vi "Switch.vi"() -> ()   [LabVIEW 2022 SP3]
uses:
  <vilib>/DAQmx/read.llb/DAQmx Read (Digital 1D Bool NChan 1Samp 1Line).vi
  <vilib>/DAQmx/miscellaneous.llb/DAQmx Fill In Error Info.vi
panel:
  out "Switches Bool":bool[](array[boolean])
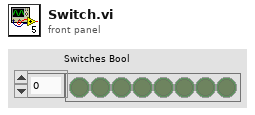
[diagram p1: front panel]
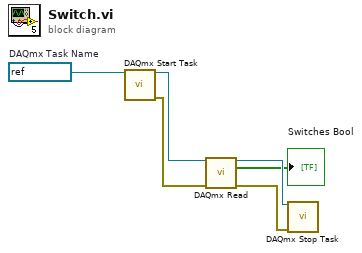
[diagram p0: block diagram]
diagram:
  w5 = refnum<k21> "Switch"  # DAQmx Task Name
  n1 = call <vilib>:"DAQmx Start Task.vi"("task/channels in"=w5) -> ("task out"=w2:refnum<k21>, "error out"=w1:errorcluster)  [unwired: 13 in]
  n2 = call-poly <vilib>:"DAQmx Read.vi"("task/channels in"=w2, "error in"=w1) -> ("task out"=w4:refnum<k21>, "data"=→"Switches Bool":bool[], "error out"=w6:errorcluster)  [unwired: 11 in]
  n3 = call <vilib>:"DAQmx Stop Task.vi"("task/channels in"=w4, "error in"=w6) -> ()  [unwired: 12 in, 2 out]
